vi "FTW-SQLite-CreateEphemeralDatabase.vi"(11 "error in":errorcluster) -> (4 "SQLite Connection":refnum<data-value>, 15 "error out":errorcluster)   [LabVIEW 2015]
uses:
  core/FTW-SQLite-Core-Structure.ctl
  core/FTW-SQLite-Core-AccessMode.ctl
  core/FTW-SQLite-Core-DatabaseType.ctl
panel:
  # "Inputs"
  # "Outputs"
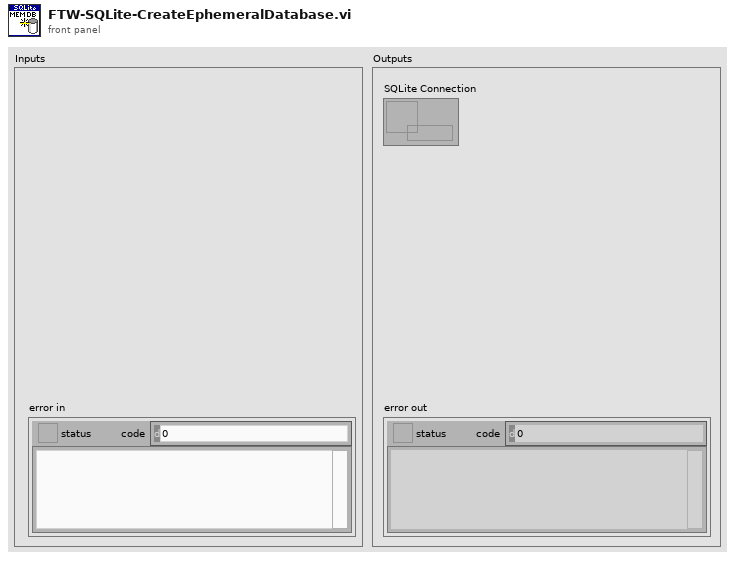
[diagram p1: front panel]
types:
  T1 = typedef "FTW-SQLite-Core-DatabaseType.ctl" = enum16{"Disk", "Memory"}
  T2 = typedef "FTW-SQLite-Core-AccessMode.ctl" = enum16{"Read", "Read/Write", "Read/Write/Create"}
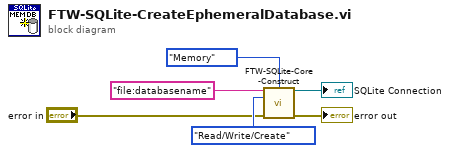
[diagram p0: block diagram]
diagram:
  n1 = call "FTW-SQLite-Core-Construct.vi"("Database URI"="file:databasename", "Database Type"=FTW-SQLite-Core-DatabaseType."Memory", "Access Mode"=FTW-SQLite-Core-AccessMode."Read/Write/Create", "error in"="error in") -> ("SQLite Connection"=→"SQLite Connection":refnum<data-value>, "error out"=→"error out":errorcluster)  [unwired: 9 in, 1 out]
